vi "LabView - Supervisory.vi"() -> ()   [LabVIEW 2018]
uses:
  <vilib>/express/express arith-compare/Formula/XNode/ExpressFormulaBlockNode.xnode
panel:
  in  "Table PWM":dbl(knob) step=1.0 scale=0.0..100.0
  in  "LastTablePWM":dbl
  out "Correction Factor %":dbl
  out "BuildingWithoutCW":dbl(graph)
  out "BuildingWithCW":dbl(graph)
  out "ResponseArray":dbl[][](array[numeric])
  # "SISTEMA DE MONITORAMENTO DO AMORTECIMENTO DE UMA ESTRUTURA ATRAVÉS DE CONTRAPESO INERCIAL"
  # "ESTRUTURA COM CONTRAPESO"
  # "FATOR DE CORREÇÃO"
  # "ESTRUTURA SEM CONTRAPESO"
  # "%"
  # "POTÊNCIA DA MESA SÍSMICA"
  # "GRUPO 7: EVERALDO JUNIOR, FABIANO MOREIRA, GABRIEL TOTOLA, PEDRO FAFÁ E RAYSSA CIBIEN"
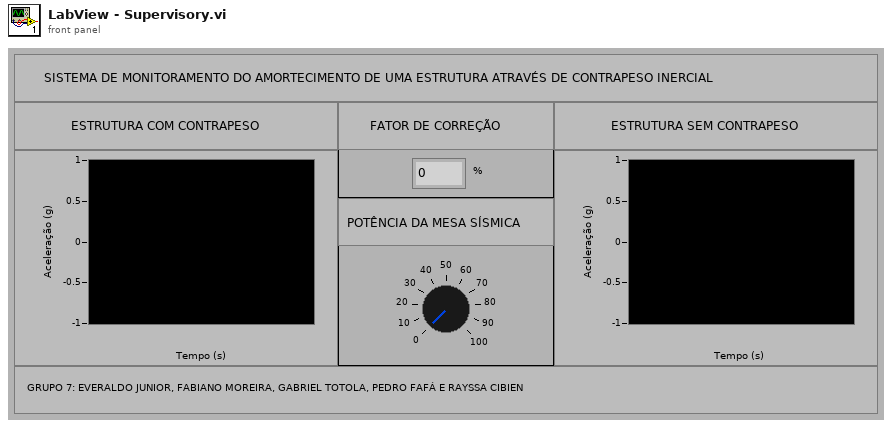
[diagram p1: front panel]
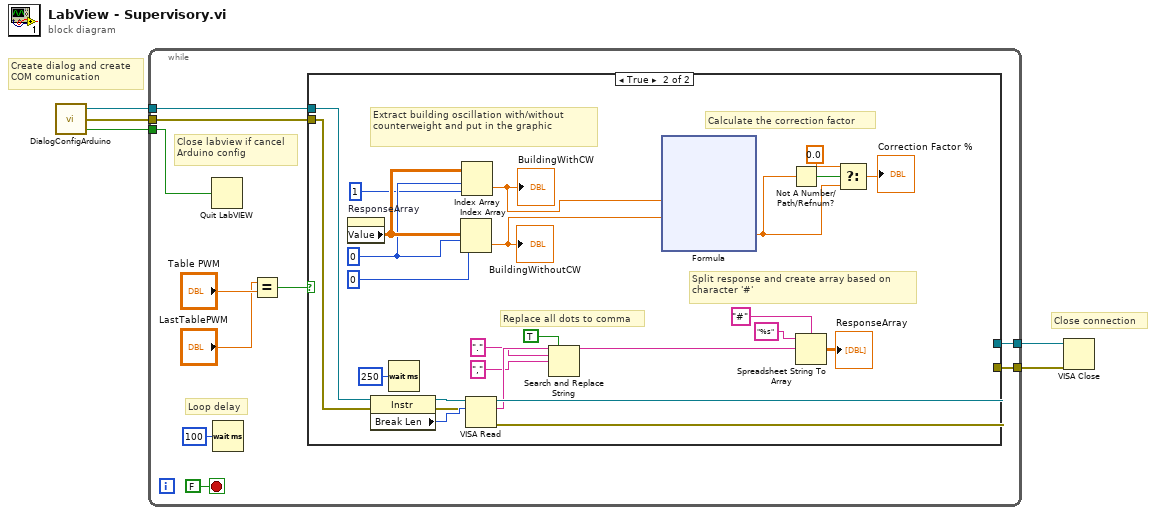
[diagram p0: block diagram]
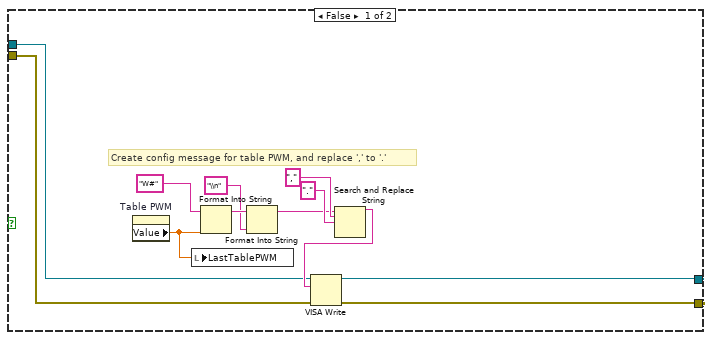
[diagram p2: hidden frame]
diagram:
  # "Create dialog and create \nCOM comunication"
  # "Close connection"
  n1 = call "DialogConfigArduino.vi"() -> ("Cancel"=w1:bool, "Error Out"=w2:errorcluster, "Port Name"=w3:refnum<visa-resource-name>)
  n2 = while {
    tunnel: w3 -> [w13]
    tunnel: w2 -> [w12]
    tunnel: [w7] -> w5
    tunnel: [w8] -> w4
    tunnel: w1 -> [w6]
    stop <- FALSE stop-if-true
    # "Close labview if cancel\nArduino config"
    # "Loop delay"
    n3 = Quit LabVIEW(quit? (T)=w6) -> ()
    n4 = Wait (ms)(milliseconds to wait=u32 100) -> ()  [unwired: 1 out]
    n5 = Equal?(x="LastTablePWM", y="Table PWM") -> (x = y?=w10:bool)
    n6 = case shown="True" w10 {
      tunnel: w13 -> [w18 w35]
      tunnel: w12 -> [w19 w36]
      tunnel: [w16 w34] -> w8
      tunnel: [w17 w33] -> w7
      frame False {
        # "Create config message for table PWM, and replace ',' to '.'"
        n7 = property on="Table PWM" class="Knob (strict)"() -> ("Value"=w25:dbl)  [unwired: 2 in, 2 out]
        n8 = local write "LastTablePWM"(w25) -> ()
        n9 = Format Into String(initial string="W#", w25) -> (resulting string=w24:string)  [unwired: 2 in, 1 out]
        n10 = Format Into String(initial string=w24, "\\n" ("search string")) -> (resulting string=w21:string)  [unwired: 2 in, 1 out]
        n11 = Search and Replace String(input string=w21, search string=",", replace string="." ("replace string (\"\")")) -> (result string=w20:string)  [unwired: 5 in, 3 out]
        n12 = VISA Write(VISA resource name=w18, write buffer=w20, error in (no error)=w19) -> (VISA resource name out=w17:refnum<visa-resource-name>, error out=w16:errorcluster)  [unwired: 1 out]
      }
      frame True {
        w42 = 0 ("index (row)")
        # "Replace all dots to comma"
        # "Calculate the correction factor"
        # "Split response and create array based on character '#'"
        # "Extract building oscillation with/without counterweight and put in the graphic"
        n13 = property on="ResponseArray" class="Arr (strict)"() -> ("Value"=w48:dbl[][])  [unwired: 2 in, 2 out]
        n14 = property class="Instr"(reference=w35, error in=w36) -> (reference out=w45:refnum<visa-resource-name>, error out=w44:errorcluster, "Break Len"=w46:i16)
        n15 = Wait (ms)(milliseconds to wait=u32 250) -> ()  [unwired: 1 out]
        n16 = Index Array(array=w48, index (row)=w42, index (col)=0 ("disabled index (col)")) -> (element=w50:dbl)
        "BuildingWithoutCW" <- w50
        n17 = Index Array(array=w48, index (row)=w42, index (col)=1) -> (element=w49:dbl)
        "BuildingWithCW" <- w49
        n18 = VISA Read(VISA resource name=w45, byte count=w46, error in (no error)=w44) -> (VISA resource name out=w33:refnum<visa-resource-name>, read buffer=w32:string, error out=w34:errorcluster)  [unwired: 1 out]
        n19 = Search and Replace String(replace all?=TRUE ("replace all? (F)"), input string=w32, search string=".", replace string="," ("replace string (\"\")")) -> (result string=w29:string)  [unwired: 4 in, 3 out]
        n20 = xnode "Formula"("WithCW"=w49, "WithoutCW"=w50) -> ("Result"=w52:dbl)  [unwired: 1 in, 1 out]
        n21 = Not A Number/Path/Refnum?(number/path/refnum=w52) -> (NaN/Path/Refnum?=w51:bool)
        n22 = Spreadsheet String To Array(delimiter (Tab)="#" ("format string"), format string="%s", spreadsheet string=w29) -> (array=→"ResponseArray":dbl[][])  [unwired: 1 in]
        n23 = Select(t=0.0, s=w51, f=w52) -> (s? t:f=→"Correction Factor %":dbl)
      }
    }
  }
  n24 = VISA Close(VISA resource name=w5, error in (no error)=w4) -> ()  [unwired: 1 out]
